vi "Binomial Random.vi"(6 "seed":i32=-1, 7 "reset":bool, 9 "p":dbl=0.02, 10 "n":i32=1, 11 "samples":i32=128) -> (0 "error":i32, 3 "binomial random data":u32[](array[numeric]))   [LabVIEW 2024, in "NI_Gmath.lvlib"]
doc: "<p>Generates random values from a variate <em>X</em>, where <em>X</em> describes the selected distribution type. You must <a href=\"nihelplauncher://docs/csh?context=lvcore_lvhowto_selectingdefaultinstpolyvi\">manually select the polymorphic instance</a> to use.</p>"
uses:
  NI_Gmath.lvlib
  NI_AALBase.lvlib
panel:
  # "Binomial Random"
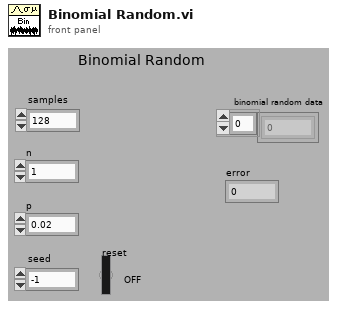
[diagram p1: front panel]
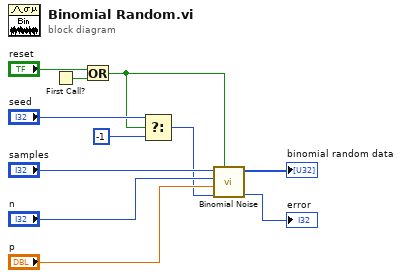
[diagram p0: block diagram]
diagram:
  n1 = First Call?() -> (First Call?: T/F=w6:bool)
  n2 = Or(x="reset", y=w6) -> (x .or. y?=w1:bool)
  n3 = Select(t="seed", s=w1, f=-1) -> (s? t:f=w2:i32)
  n4 = call "Binomial Noise.vi"("initialize?"=w1, "seed"=w2, "trial probability"="p", "trials"="n", "samples"="samples") -> ("error"=→"error":i32, "binomial noise"=→"binomial random data":u32[])  [unwired: 5 in]
